vi "GE 5565PIORC.Register.Read (U16).vi"(5 "Mask (0xFFFF)":u16=65535 format="%.0x", 7 "Address Space":T1=11 items=["VXI/VME A16"=1, "VXI/VME A24"=2, "VXI/VME A32"=3, "VXI/VME A64"=4, "PXI Memory Allocations"=9, "PXI Configuration"=10, "PXI BAR0"=11, "PXI BAR1"=12, "PXI BAR2"=13, "PXI BAR3"=14, "PXI BAR4"=15, "PXI BAR5"=16], 8 "error in (no error)":errorcluster, 10 "Offset":u32, 11 "GE 5565PIORC in":refnum<class "GE 5565PIORC.lvclass">) -> (0 "error out":errorcluster, 1 "Value":u16, 3 "GE 5565PIORC out":refnum<class "GE 5565PIORC.lvclass">)   [LabVIEW 2016, in "GE 5565PIORC.lvclass"]
uses:
  GE 5565PIORC.lvclass
  <vilib>/Instr/_visa.llb/VISA Register Access Address Space.ctl
  GE 5565PIORC.lvclass/GE 5565PIORC.ctl
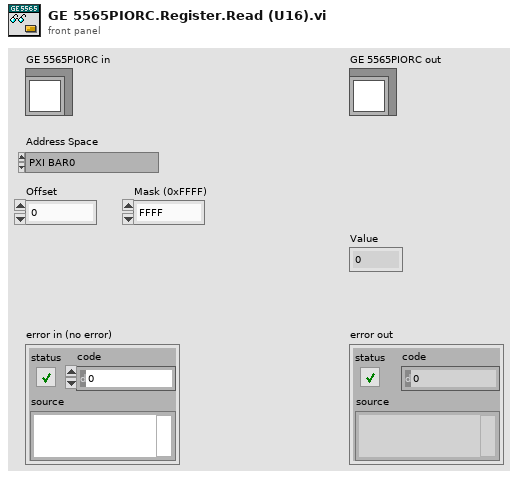
[diagram p1: front panel]
types:
  T1 = typedef "VISA Register Access Address Space.ctl" = u16
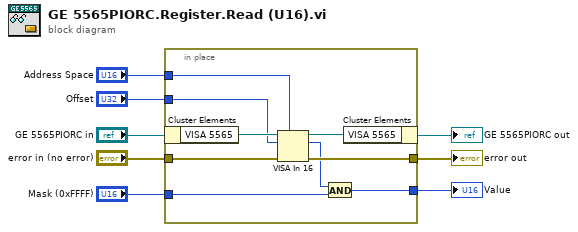
[diagram p0: block diagram]
diagram:
  n1 = in-place {
    in-place-border: "error in (no error)" -> [w15]
    in-place-border: [w14] -> w4
    in-place-border: "Address Space" -> [w13]
    in-place-border: [w11] -> w1
    in-place-border: "Mask (0xFFFF)" -> [w10]
    in-place-border: "Offset" -> [w9]
    n2 = in-place-cluster #1("GE 5565PIORC in") -> ("VISA 5565"=w17:refnum<visa-resource-name>)
    n3 = VISA In 16(7:w13, 8:w15, 10:w9, 11:w17) -> (0:w14:errorcluster, 2:w12:u16, 3:w16:refnum<visa-resource-name>)
    n4 = And(x=w12, y=w10) -> (x .and. y?=w11:u16)
    n5 = in-place-cluster #1("VISA 5565"=w16) -> (→"GE 5565PIORC out":refnum<class "GE 5565PIORC.lvclass">)
  }
  "error out" <- w4
  "Value" <- w1
